vi "VideoAccuracyCalculation.vi"(10 "AntDistance [mm]":dbl format="%_6g", 11 "AntennasPosition":u32[][](array[numeric])) -> (3 "VideoAccuracy [mm/px]":dbl format="%_6g")   [LabVIEW 2024]
uses:
  <vilib>/Analysis/baseanly.llb/Mean (DBL).vi
  <vilib>/Analysis/NI_AALBase.lvlib
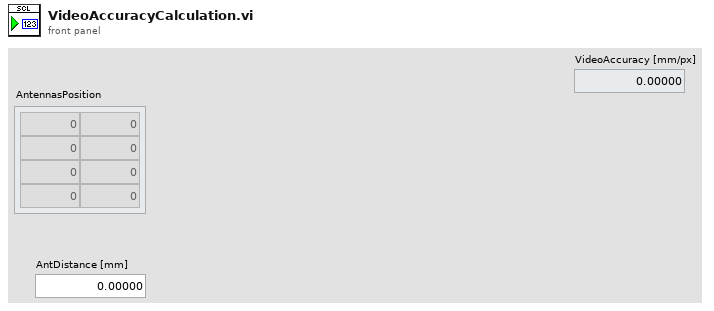
[diagram p1: front panel]
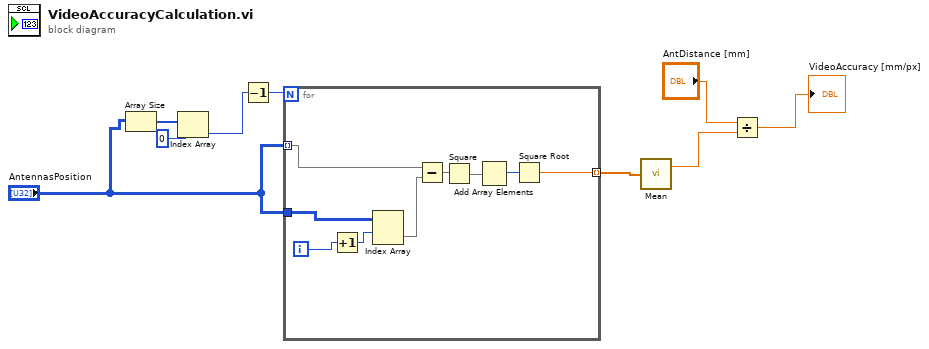
[diagram p0: block diagram]
diagram:
  n1 = Array Size(array="AntennasPosition") -> (size(s)=w8:i32[])
  n2 = Index Array(array=w8, index=0) -> (element=w5:i32)
  n3 = Decrement(x=w5) -> (x-1=w6:i32)
  n4 = for {
    N: w6 -> [_]
    tunnel: "AntennasPosition" -> [w18]
    tunnel: "AntennasPosition" -> [w14] mode=indexing
    tunnel: [w10] -> w4 mode=indexing
    i -> [w17]
    n5 = Increment(x=w17) -> (x+1=w16:i32)
    n6 = Index Array(array=w18, index (row)=w16) -> (element=w15:u32[])  [unwired: 1 in]
    n7 = Subtract(x=w14, y=w15) -> (x-y=w13:u32[])
    n8 = Square(x=w13) -> (x^2=w12:u32[])
    n9 = Add Array Elements(numeric array=w12) -> (sum=w11:u32)
    n10 = Square Root(x=w11) -> (sqrt(x)=w10:dbl)
  }
  n11 = call-poly <vilib>:"Mean.vi"("X"=w4) -> ("mean"=w2:dbl)  [unwired: 1 out]
  n12 = Divide(x="AntDistance [mm]", y=w2) -> (x/y=→"VideoAccuracy [mm/px]":dbl)
